vi "test_CSM.vi"(7 "Name (\"\" to Use UUID)":string="Event CSM Tiny") -> ()   [LabVIEW 2025]
doc: "Compact code template used to create a CSM module with a user interface. This template includes a user Event Structure for responding to user actions. The functionality of this template is identical to the CSM User Interface(UI) Module Template VI.\n\n\n> [!NOTE] <b>CSM Naming Rules</b>\n>\n> - CSM module name must be unique. Otherwise, CSM enters a `Critical Error` state.\n> - If the input module name is an empty string (\"\"), the system uses a UUID as the module name. Such a module is marked as standalone mode and does not appear in the module list.\n> - Worker Mode Rule: If the input module name ends with `#`, a worker mode node will be instantiated. Multiple worker mode nodes can form a worker mode module.\n> - Chain of Responsibility Mode Rule: If the input module name ends with `$` followed by a number, a chain of responsibility mode node will be instantiated. Multiple chain of responsibility mode nodes can form a chain of responsibility mode module.\n> - System-Level Module Rule: If the input module name starts with `.`, the module is a system-level module. Under default settings, such modules are not listed by the CSM - List Modules VI and are suitable for instantiating modules that run in the background.\n> - Submodule Rule: `.` is also allowed in a module name to separate the module name into multiple parts. CSM does not have strict rules for submodules. The `.` in the module name only marks the logical relationship between different modules. From an execution perspective, they are considered independent modules. The only difference is that you can obtain a list of logical submodules via the CSM - List Submodules VI.\n\n\n-- <b>Controls</b> --\n- <b>Name (\"\" to use UUID)</b>: CSM module name. Refer to <b>CSM Naming Rules</b> for module naming rules."
uses:
  <userlib>/_NEVSTOP/Communicable State Machine(CSM)/AdvanceAPI/CSM - Revert Arguments-Safe String.vi
  <userlib>/_NEVSTOP/Communicable State Machine(CSM)/_Shared/Trim Single-line Text.vi
  <userlib>/_NEVSTOP/Communicable State Machine(CSM)/AdvanceAPI/CSM - Break Down Multiple States String.vi
  <userlib>/_NEVSTOP/Communicable State Machine(CSM)/AdvanceAPI/CSM - Compact Multiple States.vi
  <userlib>/_NEVSTOP/Communicable State Machine(CSM)/AdvanceAPI/CSM - Make String Arguments Safe.vi
  <userlib>/_NEVSTOP/Communicable State Machine(CSM)/AdvanceAPI/CSM - Keywords.vi
  <userlib>/_NEVSTOP/Communicable State Machine(CSM)/Communicable State Machine.lvlib
panel:
  out "State History":string
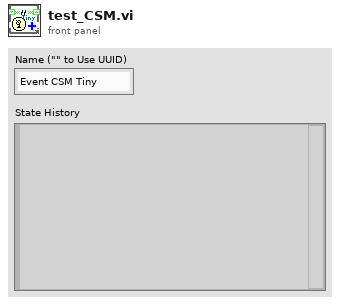
[diagram p1: front panel]
types:
  T1 = enum32{"Invalid", "Standard", "Closed", "Hidden", "Minimized", "Maximized"}
  T2 = enum32{"invalid app kind", "Development System", "Run Time System", "Student Edition", "Embedded LabVIEW", "Evaluation", "Custom"}
  T3 = typedef "Communicable State Machine.lvlib/_CSM_Response Source Message.ctl" = cluster{"‘State":string, "’Arguments":string, "’Error":errorcluster}
  T4 = cluster{"Current VI Reference":refnum<vi>, "Close Panel on Exit?":bool}
  T5 = cluster{"Core":cluster{"Current VI Reference":refnum<vi>, "Close Panel on Exit?":bool}, "Your Boolean data":bool, "Your string data":string}
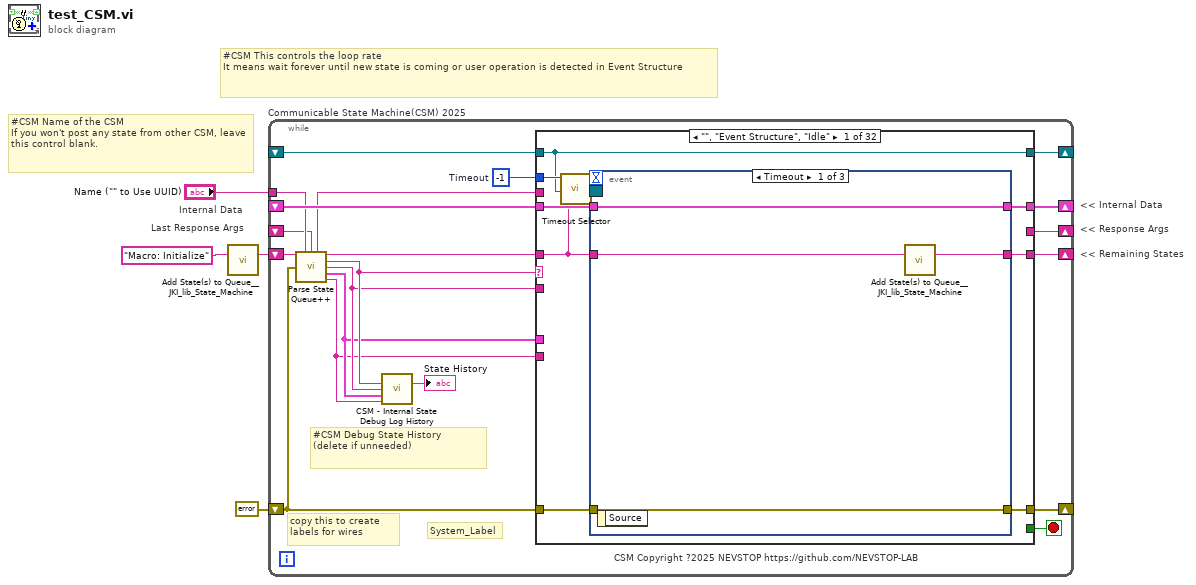
[diagram p0: block diagram]
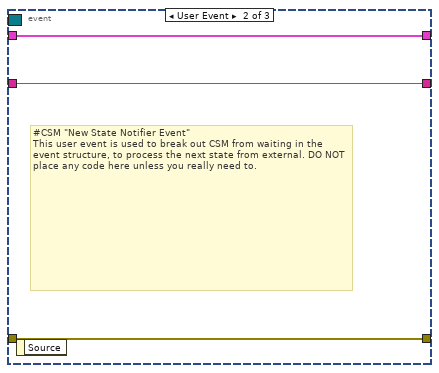
[diagram p2: hidden frame]
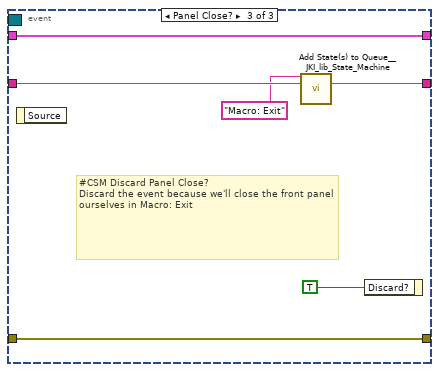
[diagram p3: hidden frame]
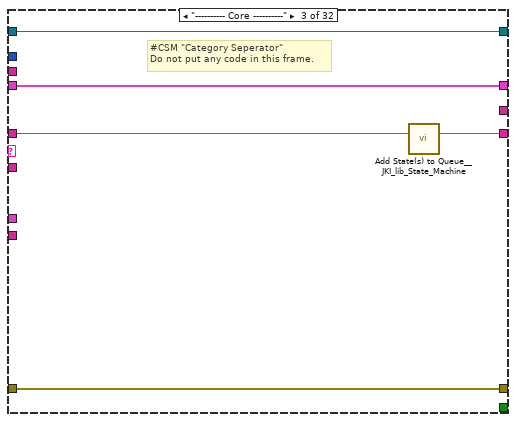
[diagram p5: hidden frame]
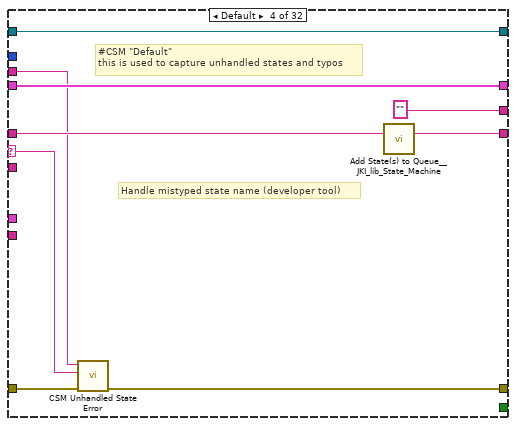
[diagram p6: hidden frame]
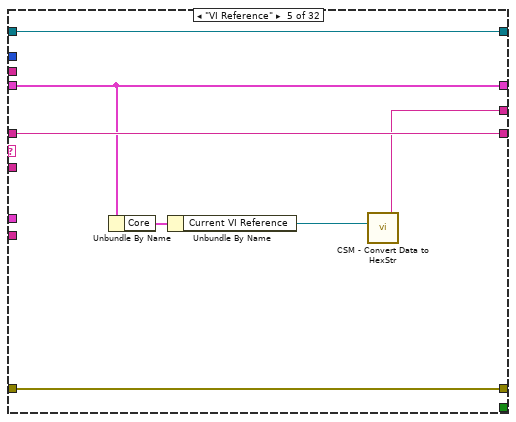
[diagram p7: hidden frame]
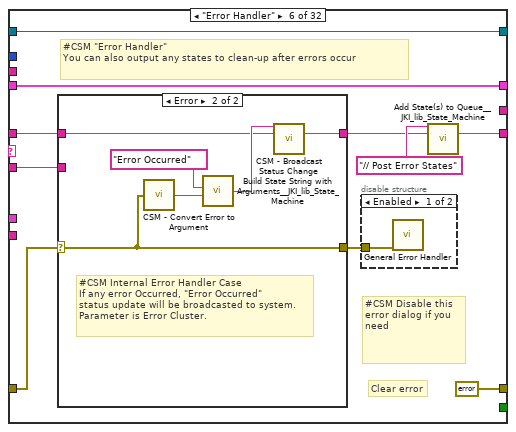
[diagram p8: hidden frame]
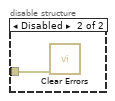
[diagram p9: hidden frame]
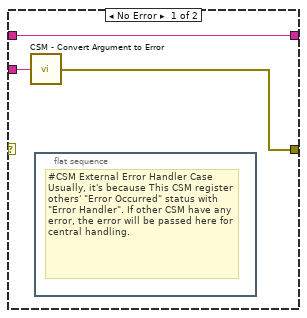
[diagram p10: hidden frame]
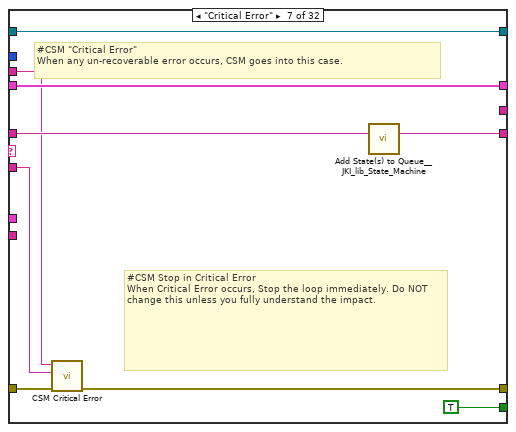
[diagram p11: hidden frame]
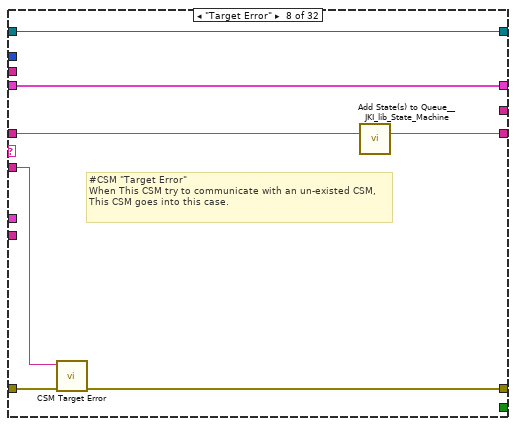
[diagram p12: hidden frame]
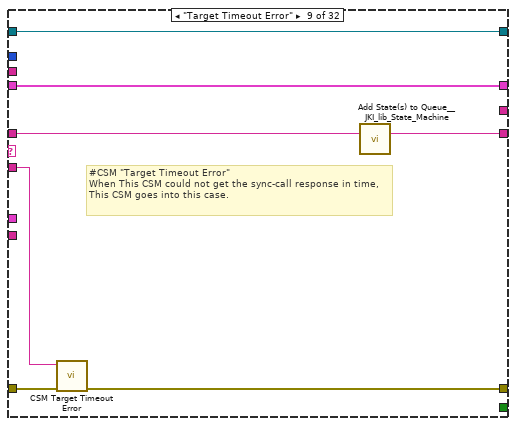
[diagram p13: hidden frame]
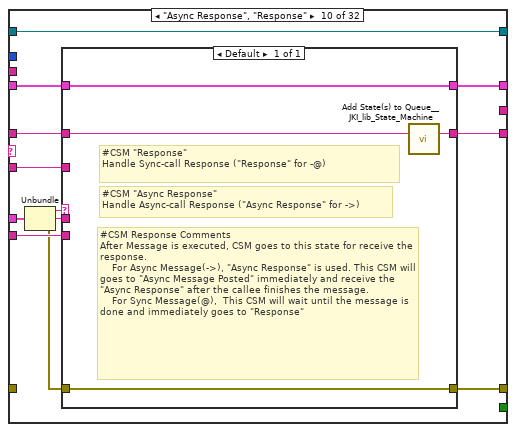
[diagram p14: hidden frame]
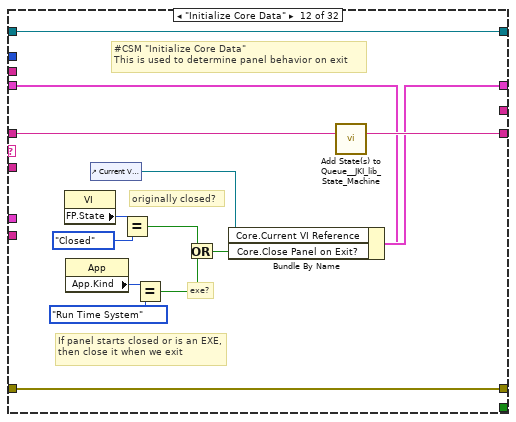
[diagram p16: hidden frame]
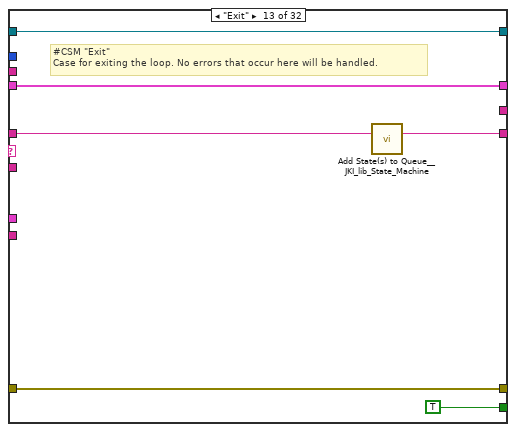
[diagram p17: hidden frame]
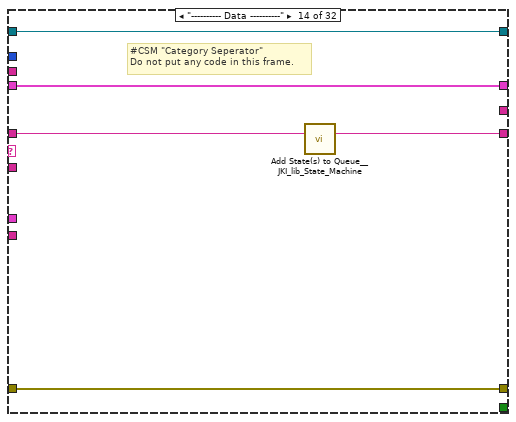
[diagram p18: hidden frame]
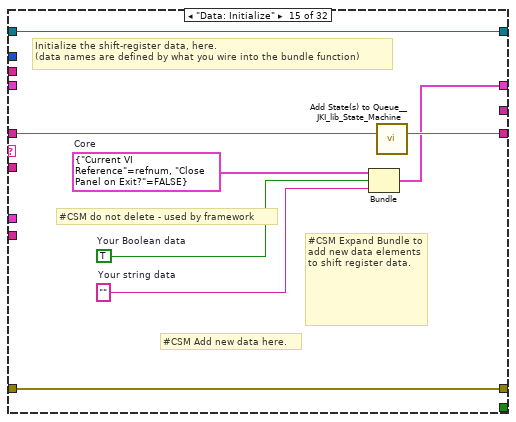
[diagram p19: hidden frame]
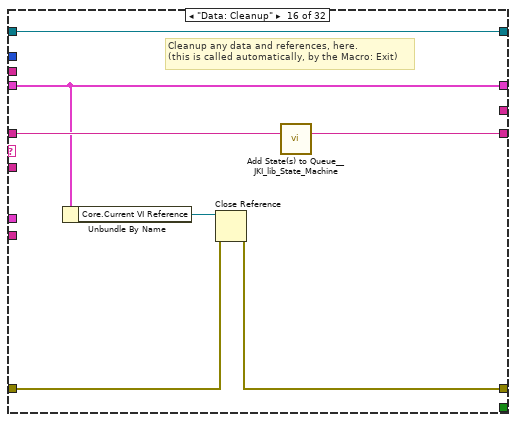
[diagram p20: hidden frame]
diagram:
  # "Last Response Args"
  # "Internal Data"
  # "#CSM Name of the CSM\nIf you won't post any state from other CSM, leave this control blank."
  # "#CSM This controls the loop rate\nIt means wait forever until new state is coming or user operation is detected in Event Structure"
  # "<< Internal Data"
  # "<< Response Args"
  # "<< Remaining States"
  n1 = call <vilib>:"Add State(s) to Queue__JKI_lib_State_Machine.vi"("State(s) in (\"\")"="Macro: Initialize" ("Init State(\"Macro: Initialize\")")) -> ("States Out"=w4:string)  [unwired: 14 in]
  n2 = while "Communicable State Machine(CSM) 2025" {
    shift-right: [w19] -> _
    shift-left: _ -> [w18]
    shift-right: [w22] -> _
    shift-left: errorcluster {"status"=FALSE, "code"=0, "source"=""} ("error out") -> [w16]
    shift-right: [w21] -> _
    shift-left: w4 -> [w23]
    tunnel: "Name (\"\" to Use UUID)" -> [w12]
    shift-right: [w15] -> _
    shift-left: _ -> [w6]
    shift-right: [w14] -> _
    shift-left: _ -> [w13]
    stop <- w20 stop-if-true
    w17 = -1  # Timeout
    # "#CSM Debug State History\n(delete if unneeded)"
    # "copy this to create labels for wires"
    # "System_Label"
    # "CSM Copyright ?2025 NEVSTOP https://github.com/NEVSTOP-LAB"
    n3 = call <userlib>:"Parse State Queue++.vi"("State Queue"=w23, "Name (\"\" to Use UUID)"=w12, "Response Arguments"=w6, "Previous Error"=w16) -> ("Name Used"=w7:string, "Remaining States"=w24:string, "Current State"=w11:string, "Arguments"=w10:string, "Additional Information"=w9:T3, "Source CSM"=w8:string)  [unwired: 6 in]
    n4 = call <userlib>:"CSM - Internal State Debug Log History.vi"("State"=w11, "Arguments (\"\")"=w10, ">> Response Source Message >>"=w9, "Source (\"\")"=w8) -> ("Debug Log"=→"State History":string)  [unwired: 11 in]
    n5 = case shown="\"\", \"Event Structure\", \"Idle\"" w11 {
      selector: w11 -> [_ _ _ w58 _ _ _ _ _ _ _ _ _ _ _ _ _ _ _ _ _ _ _ _ _ _ _ _ _ _ _ _]
      tunnel: w24 -> [w25 w49 w55 w63 w70 w76 w99 w105 w112 w121 w134 w149 w155 w160 w168 w175 w180 w187 w191 w197 w202 w209 w225 w295 w301 w313 w316 w321 w327 w335 w340 w345]
      tunnel: w10 -> [_ _ _ _ _ w75 w94 w104 w111 w120 _ _ _ _ _ _ _ _ _ _ _ w204 w219 _ _ _ _ _ w324 _ _ _]
      tunnel: w18 -> [w32 w48 w52 w61 w69 w80 w100 w107 w114 w123 w133 w142 w153 w157 _ w170 w177 w186 w190 w194 w200 w207 w221 w292 w298 w310 w315 w320 w326 w332 w337 w342]
      tunnel: [w31 w50 w53 w56 w71 errorcluster {"status"=FALSE, "code"=0, "source"=""} ("error out") w95 w102 w109 w126 w135 w146 w152 w158 w165 w171 w178 w181 w189 w195 w199 w205 w222 w293 w299 w311 w317 w322 w328 w333 w338 w343] -> w22
      tunnel: w16 -> [w30 w50 w53 w64 w71 w77 w101 w103 w110 _ w135 w146 w152 w158 w165 w172 w178 _ w192 w195 w199 w206 w223 w293 w299 w311 w317 w322 w328 w333 w338 w343]
      tunnel: [w33 w49 w54 w62 w70 w72 w98 w108 w115 w122 w134 w148 w154 w159 w167 w174 w179 w187 w191 w196 w201 w208 w224 w294 w300 w312 w316 w321 w327 w334 w339 w344] -> w21
      tunnel: [_ _ _ _ _ _ TRUE _ _ _ _ _ TRUE _ _ _ _ _ _ _ _ _ _ _ _ _ _ _ _ _ _ _] -> w20
      tunnel: [w29 w48 w52 w61 w69 w80 w100 w107 w114 w124 w133 w147 w153 w157 w166 w170 w177 w186 w190 w194 w200 w207 w221 w292 w298 w310 w315 w320 w326 w332 w337 w342] -> w19
      tunnel: w17 -> [w28 _ _ _ _ _ _ _ _ _ _ _ _ _ _ _ _ _ _ _ _ _ _ _ _ _ _ _ _ _ _ _]
      tunnel: w8 -> [_ _ _ _ _ _ _ _ _ w118 _ _ _ _ _ _ _ _ _ _ _ _ _ _ _ _ _ _ _ _ _ _]
      tunnel: w9 -> [_ _ _ _ _ _ _ _ _ w125 _ _ _ _ _ _ _ _ _ _ _ _ _ _ _ _ _ _ _ _ _ _]
      tunnel: [_ _ _ "" w65 _ _ _ _ _ _ _ _ _ _ _ _ _ _ _ _ _ _ _ _ _ _ "API1 Response" w323 _ _ _] -> w15
      tunnel: [w27 w47 w51 w59 w68 w79 w96 w106 w113 w127 w132 w136 w150 w156 w161 w169 w176 w185 w188 w193 w198 w203 w218 w291 w296 w303 w314 w319 w325 w331 w336 w341] -> w14
      tunnel: w13 -> [w27 w47 w51 w59 w68 w79 w96 w106 w113 w127 w132 w136 w150 w156 w161 w169 w176 _ w188 w193 w198 w203 w218 w291 w296 w303 w314 w319 w325 w331 w336 w341]
      tunnel: w7 -> [_ _ _ w57 _ _ w93 _ _ _ _ _ _ _ _ _ _ w184 _ _ _ _ _ _ _ _ _ _ _ _ _ _]
      frame "", "Event Structure", "Idle" {
        n6 = call <userlib>:"Timeout Selector.vi"("Remaining States"=w25, "Timeout Expected"=w28) -> ("Timeout"=w26:i32)  [unwired: 5 in]
        n7 = event shown="[0] Timeout" {
          selector: w27 -> [_ _ _]
          dyn-events: _ -> [_ _ _]
          timeout: w26 -> [_ _ _]
          tunnel: w25 -> [w37 w39 w46]
          tunnel: [w36 w39 w45] -> w33
          tunnel: w32 -> [w34 w40 w43]
          tunnel: [w35 w38 w44] -> w31
          tunnel: w30 -> [w35 w38 w44]
          tunnel: [w34 w40 w43] -> w29
          event Timeout {
            n8 = event-data() -> ()  [unwired: 1 in, 1 out]
            n9 = call <vilib>:"Add State(s) to Queue__JKI_lib_State_Machine.vi"("State(s) in (\"\")"=w37) -> ("States Out"=w36:string)  [unwired: 14 in]
          }
          event User Event {
            # "#CSM \"New State Notifier Event\"\nThis user event is used to break out CSM from waiting in the event structure, to process the next state from external. DO NOT place any code here unless you really need to."
            n10 = event-data() -> ()  [unwired: 1 in, 1 out]
          }
          event Panel Close? {
            # "#CSM Discard Panel Close?\nDiscard the event because we'll close the front panel ourselves in Macro: Exit"
            n11 = event-data() -> ()  [unwired: 1 in, 1 out]
            n12 = call <vilib>:"Add State(s) to Queue__JKI_lib_State_Machine.vi"("State(s) in Front (\"\")"="Macro: Exit", "State(s) in (\"\")"=w46) -> ("States Out"=w45:string)  [unwired: 13 in]
            n13 = event-data("Discard?"=TRUE) -> ()  [unwired: 1 in, 1 out]
          }
        }
      }
      frame "CSM Documentation" {
        # "#CSM README FIRST\n\nCommunicable State Machine(CSM) is a LabVIEW application framework that builds upon JKI State Machine(JKISM). It follows the pattern of JKISM and extends the keywords to describe message communication between modules, including concepts such as Sync-Message, Async-Message, Subscription/Unsubscription of status - essential elements for creating reusable code modules. For more information, please visit the CSM wiki: https://nevstop-lab.github.io/CSM-Wiki/\n\nFor instructions on JKI State Machine, visit: http://jki.net/state-machine/\nFor information about CSM, visit: https://github.com/NEVSTOP-LAB"
        # "#CSM \"Documentation\"\nCase for holding CSM Documenation"
      }
      frame "---------- Core ----------" {
        # "#CSM \"Category Seperator\"\nDo not put any code in this frame."
        n14 = call <vilib>:"Add State(s) to Queue__JKI_lib_State_Machine.vi"("State(s) in (\"\")"=w55) -> ("States Out"=w54:string)  [unwired: 14 in]
      }
      frame Default {
        # "#CSM \"Default\"\nthis is used to capture unhandled states and typos"
        # "Handle mistyped state name (developer tool)"
        n15 = call <userlib>:"CSM Unhandled State Error.vi"("error in (no error)"=w64, "Undefined State"=w58, "CSM Name"=w57) -> ("error out"=w56:errorcluster)  [unwired: 8 in]
        n16 = call <vilib>:"Add State(s) to Queue__JKI_lib_State_Machine.vi"("State(s) in (\"\")"=w63) -> ("States Out"=w62:string)  [unwired: 14 in]
      }
      frame "VI Reference" {
        n17 = Unbundle By Name(w69) -> ("Core"=w67:T4)
        n18 = Unbundle By Name(w67) -> ("Current VI Reference"=w66:refnum<vi>)
        n19 = call <userlib>:"CSM - Convert Data to HexStr.vi"("Variant"=w66) -> ("HEX String (0-9,A-F)"=w65:string)  [unwired: 8 in]
      }
      frame "Error Handler" {
        # "#CSM Disable this error dialog if you need"
        # "#CSM \"Error Handler\"\nYou can also output any states to clean-up after errors occur"
        # "Clear error"
        n20 = case shown="Error" w77 {
          selector: w77 -> [_ w87]
          tunnel: [w86 w89] -> w73
          tunnel: w76 -> [w86 w88]
          tunnel: w75 -> [w85 _]
          tunnel: [w84 w87] -> w78
          frame No Error {
            n21 = call <userlib>:"CSM - Convert Argument to Error.vi"("Argument"=w85) -> ("Error"=w84:errorcluster)  [unwired: 4 in]
            n22 = flat-sequence {
              frame #0 {
                # "#CSM External Error Handler Case\nUsually, it's because This CSM register others' \"Error Occurred\" status with \"Error Handler\". If other CSM have any error, the error will be passed here for central handling."
              }
            }
          }
          frame Error {
            # "#CSM Internal Error Handler Case \nIf any error Occurred, \"Error Occurred\" \nstatus update will be broadcasted to system.\nParameter is Error Cluster."
            n23 = call <userlib>:"CSM - Convert Error to Argument.vi"("Error"=w87) -> ("Argument"=w91:string)  [unwired: 4 in]
            n24 = call <vilib>:"Build State String with Arguments__JKI_lib_State_Machine.vi"("Arguments (\"\")"=w91, "State"="Error Occurred" ("Status with Arguments")) -> ("State with Arguments"=w90:string)  [unwired: 4 in]
            n25 = call <userlib>:"CSM - Broadcast Status Change.vi"("Status With Arguments"=w90, "State Queue"=w88) -> ("Remaining States"=w89:string)  [unwired: 13 in]
          }
        }
        n26 = disable-structure shown="Enabled" {
          disable-tunnel: w78 -> [w82 w83]
          frame Enabled {
            n27 = call <vilib>:"General Error Handler.vi"("error in (no error)"=w82) -> ()  [unwired: 10 in, 5 out]
          }
          frame Disabled {
            n28 = call <vilib>:"Clear Errors.vi"("error in (no error)"=w83) -> ()  [unwired: 5 in, 2 out]
          }
        }
        n29 = call <vilib>:"Add State(s) to Queue__JKI_lib_State_Machine.vi"("State(s) in Front (\"\")"="// Post Error States", "State(s) in (\"\")"=w73) -> ("States Out"=w72:string)  [unwired: 13 in]
      }
      frame "Critical Error" {
        # "#CSM Stop in Critical Error\nWhen Critical Error occurs, Stop the loop immediately. Do NOT change this unless you fully understand the impact."
        # "#CSM \"Critical Error\"\nWhen any un-recoverable error occurs, CSM goes into this case."
        n30 = call <userlib>:"CSM Critical Error.vi"("error in (no error)"=w101, "Arugments (As Reason)"=w94, "CSM Name"=w93) -> ("error out"=w95:errorcluster)  [unwired: 8 in]
        n31 = call <vilib>:"Add State(s) to Queue__JKI_lib_State_Machine.vi"("State(s) in (\"\")"=w99) -> ("States Out"=w98:string)  [unwired: 14 in]
      }
      frame "Target Error" {
        # "#CSM \"Target Error\"\nWhen This CSM try to communicate with an un-existed CSM, This CSM goes into this case."
        n32 = call <userlib>:"CSM Target Error.vi"("error in (no error)"=w103, "Arguments (As CSM Name)"=w104) -> ("error out"=w102:errorcluster)  [unwired: 9 in]
        n33 = call <vilib>:"Add State(s) to Queue__JKI_lib_State_Machine.vi"("State(s) in (\"\")"=w105) -> ("States Out"=w108:string)  [unwired: 14 in]
      }
      frame "Target Timeout Error" {
        # "#CSM \"Target Timeout Error\"\nWhen This CSM could not get the sync-call response in time, This CSM goes into this case."
        n34 = call <userlib>:"CSM Target Timeout Error.vi"("error in (no error)"=w110, "Arguments (As CSM Name)"=w111) -> ("error out"=w109:errorcluster)  [unwired: 9 in]
        n35 = call <vilib>:"Add State(s) to Queue__JKI_lib_State_Machine.vi"("State(s) in (\"\")"=w112) -> ("States Out"=w115:string)  [unwired: 14 in]
      }
      frame "Async Response", "Response" {
        n36 = Unbundle(w125) -> ("‘State"=w119:string, "’Arguments"=w117:string, "’Error"=w116:errorcluster)
        n37 = case shown="Default" w119 {
          tunnel: [w131] -> w126
          tunnel: w116 -> [w131]
          tunnel: [w130] -> w124
          tunnel: w123 -> [w130]
          tunnel: [w128] -> w122
          tunnel: w121 -> [w129]
          tunnel: w120 -> [_]
          tunnel: w118 -> [_]
          tunnel: w117 -> [_]
          frame Default {
            # "#CSM Response Comments\nAfter Message is executed, CSM goes to this state for receive the response.\n    For Async Message(->), \"Async Response\" is used. This CSM will goes to \"Async Message Posted\" immediately and receive the \"Async Response\" after the callee finishes the message.\n    For Sync Message(@),  This CSM will wait until the message is done and immediately goes to \"Response\""
            # "#CSM \"Async Response\"\nHandle Async-call Response (\"Async Response\" for ->)"
            # "#CSM \"Response\"\nHandle Sync-call Response (\"Response\" for -@)"
            n38 = call <vilib>:"Add State(s) to Queue__JKI_lib_State_Machine.vi"("State(s) in (\"\")"=w129) -> ("States Out"=w128:string)  [unwired: 14 in]
          }
        }
      }
      frame "Async Message Posted" {
        # "#CSM \"Async Message Posted\"\nAfter Async Message is posted (-> or ->| ), CSM goes to this state for post-action.\nYou can use Argument - State to tell which Async Message is called."
      }
      frame "Initialize Core Data" {
        # "#CSM \"Initialize Core Data\"\nThis is used to determine panel behavior on exit"
        # "originally closed?"
        # "exe?"
        # "If panel starts closed or is an EXE, then close it when we exit"
        n39 = property class="VI"() -> ("FP.State"=w139:T1)  [unwired: 2 in, 2 out]
        n40 = property class="App"() -> ("App.Kind"=w145:T2)  [unwired: 2 in, 2 out]
        n41 = control-ref of="Current VI Reference"() -> (w140:refnum<vi>)
        n42 = Equal?(x=w139, y=T1."Closed" ("Front Panel Window:State")) -> (x = y?=w137:bool)
        n43 = Equal?(x=w145, y=T2."Run Time System" ("Application:Kind")) -> (x = y?=w143:bool)
        n44 = Or(x=w137, y=w143) -> (x .or. y?=w141:bool)
        n45 = Bundle By Name(cluster=w142, "Core.Current VI Reference"=w140, "Core.Close Panel on Exit?"=w141) -> (w147:T5)
        n46 = call <vilib>:"Add State(s) to Queue__JKI_lib_State_Machine.vi"("State(s) in (\"\")"=w149) -> ("States Out"=w148:string)  [unwired: 14 in]
      }
      frame "Exit" {
        # "#CSM \"Exit\"\nCase for exiting the loop. No errors that occur here will be handled."
        n47 = call <vilib>:"Add State(s) to Queue__JKI_lib_State_Machine.vi"("State(s) in (\"\")"=w155) -> ("States Out"=w154:string)  [unwired: 14 in]
      }
      frame "---------- Data ----------" {
        # "#CSM \"Category Seperator\"\nDo not put any code in this frame."
        n48 = call <vilib>:"Add State(s) to Queue__JKI_lib_State_Machine.vi"("State(s) in (\"\")"=w160) -> ("States Out"=w159:string)  [unwired: 14 in]
      }
      frame "Data: Initialize" {
        w162 = T4 {"Current VI Reference"=refnum, "Close Panel on Exit?"=FALSE}  # Core
        w164 = TRUE  # Your Boolean data
        w163 = ""  # Your string data
        # "#CSM do not delete - used by framework"
        # "#CSM Expand Bundle to add new data elements to shift register data."
        # "#CSM Add new data here."
        # "Initialize the shift-register data, here.\n(data names are defined by what you wire into the bundle function)"
        n49 = Bundle("Core"=w162, "Your Boolean data"=w164, "Your string data"=w163) -> (w166:T5)  [unwired: 1 in]
        n50 = call <vilib>:"Add State(s) to Queue__JKI_lib_State_Machine.vi"("State(s) in (\"\")"=w168) -> ("States Out"=w167:string)  [unwired: 14 in]
      }
      frame "Data: Cleanup" {
        # "Cleanup any data and references, here.\n(this is called automatically, by the Macro: Exit)"
        n51 = Unbundle By Name(w170) -> ("Core.Current VI Reference"=w173:refnum<vi>)
        n52 = Close Reference(reference=w173, error in (no error)=w172) -> (error out=w171:errorcluster)
        n53 = call <vilib>:"Add State(s) to Queue__JKI_lib_State_Machine.vi"("State(s) in (\"\")"=w175) -> ("States Out"=w174:string)  [unwired: 14 in]
      }
      frame "---------- Events ----------" {
        # "#CSM \"Category Seperator\"\nDo not put any code in this frame."
        n54 = call <vilib>:"Add State(s) to Queue__JKI_lib_State_Machine.vi"("State(s) in (\"\")"=w180) -> ("States Out"=w179:string)  [unwired: 14 in]
      }
      frame "Events: Register" {
        # "#CSM \"Events: Register\"\nRegister user event. New Message Event is registered to break CSM waiting in event structure by default."
        # "#CSM Register New Message Event\nRegister message event to break Waiting in Event structure."
        n55 = call <userlib>:"CSM - Get New State Notifier Event.vi"("Name (\"\" to Use UUID)"=w184) -> ("error out"=w182:errorcluster, "New State Notifier Event"=w183:refnum<user-event>)  [unwired: 9 in]
        n56 = register-events(error in=w182, w183) -> (reference out=w185:refnum<event-registration>, error out=w181:errorcluster)  [unwired: 1 in]
      }
      frame "Events: Unregister" {
        # "#CSM \"Events: Unregister\"\nUnregister user event."
        n57 = Unregister For Events(event registration refnum=w188, error in=w192) -> (error out=w189:errorcluster)
      }
      frame "---------- UI ----------" {
        # "#CSM \"Category Seperator\"\nDo not put any code in this frame."
        n58 = call <vilib>:"Add State(s) to Queue__JKI_lib_State_Machine.vi"("State(s) in (\"\")"=w197) -> ("States Out"=w196:string)  [unwired: 14 in]
      }
      frame "UI: Initialize" {
        # "#CSM \"UI: Initialize\"\nInitialize the User Interface, here.\n(this is called automatically, by the Macro: Init)"
        n59 = call <vilib>:"Add State(s) to Queue__JKI_lib_State_Machine.vi"("State(s) in (\"\")"=w202) -> ("States Out"=w201:string)  [unwired: 14 in]
      }
      frame "UI: Cursor Set" {
        # "#CSM \"UI: Cursor Set\"\nSet and Unset Cursor Busy.\n(Usage: \"UI: Cursor Set >> Busy|Idle\")"
        # "Argument"
        n60 = disable-structure shown="Default" {
          disable-tunnel: w206 -> [w212 w217]
          disable-tunnel: [w211 w217] -> w205
          disable-tunnel: w204 -> [w210 _]
          frame condition #0 (active) {
            n61 = case shown="\"Idle\", Default" w210 {
              tunnel: w212 -> [w214 w216]
              tunnel: [w213 w215] -> w211
              frame "Idle", Default {
                n62 = call <vilib>:"Unset Busy.vi"("error in (no error)"=w214) -> ("error out"=w213:errorcluster)  [unwired: 10 in]
              }
              frame "Busy" {
                n63 = call <vilib>:"Set Busy.vi"("error in (no error)"=w216) -> ("error out"=w215:errorcluster)  [unwired: 9 in, 1 out]
              }
            }
          }
          frame condition #1 {
          }
        }
        n64 = call <vilib>:"Add State(s) to Queue__JKI_lib_State_Machine.vi"("State(s) in (\"\")"=w209) -> ("States Out"=w208:string)  [unwired: 14 in]
      }
      frame "UI: Front Panel State" {
        # "#CSM \"UI: Front Panel State\"\nSet Front Panel Open or Closed\n(Usage: \"UI: Front Panel State >> Open|Close\")"
        # "Argument"
        n65 = Unbundle By Name(w221) -> ("Core.Current VI Reference"=w220:refnum<vi>)
        n66 = call <vilib>:"Add State(s) to Queue__JKI_lib_State_Machine.vi"("State(s) in (\"\")"=w225) -> ("States Out"=w224:string)  [unwired: 14 in]
        n67 = case shown="\"Close\", \"Closed\"" w219 {
          tunnel: w223 -> [w231 w246 w257 w270 w283]
          tunnel: [w233 w247 w259 w272 w285] -> w222
          tunnel: w220 -> [w232 w244 w258 w271 w284]
          frame "Open", "Standard", Default {
            w226 = T1."Standard" ("State")
            n68 = property class="VI"(reference=w232, error in=w231) -> (reference out=w229:refnum<vi>, error out=w230:errorcluster, "FP.State"=w228:T1)
            n69 = Not Equal?(x=w228, y=w226) -> (x != y?=w227:bool)
            n70 = case shown="True" w227 {
              tunnel: [w237 w239] -> w233
              tunnel: w230 -> [w236 w239]
              tunnel: w229 -> [w235 _]
              tunnel: w226 -> [w234 _]
              frame True {
                n71 = invoke class="VI" method="FP.Open"(reference=w235, error in=w236, "Activate"=TRUE, "State"=w234) -> (error out=w237:errorcluster)  [unwired: 1 in, 4 out]
              }
              frame False {
              }
            }
          }
          frame "Close", "Closed" {
            n72 = property class="VI"(reference=w244, error in=w246) -> (reference out=w243:refnum<vi>, error out=w245:errorcluster, "FP.State"=w241:T1)
            n73 = Not Equal?(x=w241, y=T1."Closed" ("Front Panel Window:State")) -> (x != y?=w240:bool)
            n74 = case shown="False" w240 {
              tunnel: [w248 w251] -> w247
              tunnel: w245 -> [w248 w250]
              tunnel: w243 -> [_ w249]
              frame False {
              }
              frame True {
                n75 = invoke class="VI" method="FP.Close"(reference=w249, error in=w250) -> (error out=w251:errorcluster)  [unwired: 1 in, 2 out]
              }
            }
          }
          frame "Hidden", "Hide" {
            w252 = T1."Hidden" ("State")
            n76 = property class="VI"(reference=w258, error in=w257) -> (reference out=w255:refnum<vi>, error out=w256:errorcluster, "FP.State"=w254:T1)
            n77 = Not Equal?(x=w254, y=w252) -> (x != y?=w253:bool)
            n78 = case shown="True" w253 {
              tunnel: [w263 w264] -> w259
              tunnel: w256 -> [w262 w264]
              tunnel: w255 -> [w261 _]
              tunnel: w252 -> [w260 _]
              frame True {
                n79 = invoke class="VI" method="FP.Open"(reference=w261, error in=w262, "State"=w260) -> (error out=w263:errorcluster)  [unwired: 2 in, 4 out]
              }
              frame False {
              }
            }
          }
          frame "Minimize", "Minimized" {
            w265 = T1."Minimized" ("State")
            n80 = property class="VI"(reference=w271, error in=w270) -> (reference out=w268:refnum<vi>, error out=w269:errorcluster, "FP.State"=w267:T1)
            n81 = Not Equal?(x=w267, y=w265) -> (x != y?=w266:bool)
            n82 = case shown="True" w266 {
              tunnel: [w276 w277] -> w272
              tunnel: w269 -> [w275 w277]
              tunnel: w268 -> [w274 _]
              tunnel: w265 -> [w273 _]
              frame True {
                n83 = invoke class="VI" method="FP.Open"(reference=w274, error in=w275, "State"=w273) -> (error out=w276:errorcluster)  [unwired: 2 in, 4 out]
              }
              frame False {
              }
            }
          }
          frame "Maximize", "Maximized" {
            w278 = T1."Maximized" ("State")
            n84 = property class="VI"(reference=w284, error in=w283) -> (reference out=w281:refnum<vi>, error out=w282:errorcluster, "FP.State"=w280:T1)
            n85 = Not Equal?(x=w280, y=w278) -> (x != y?=w279:bool)
            n86 = case shown="True" w279 {
              tunnel: [w289 w290] -> w285
              tunnel: w282 -> [w288 w290]
              tunnel: w281 -> [w287 _]
              tunnel: w278 -> [w286 _]
              frame True {
                n87 = invoke class="VI" method="FP.Open"(reference=w287, error in=w288, "State"=w286) -> (error out=w289:errorcluster)  [unwired: 2 in, 4 out]
              }
              frame False {
              }
            }
          }
        }
      }
      frame "---------- Macro ----------" {
        # "#CSM \"Category Seperator\"\nDo not put any code in this frame."
        n88 = call <vilib>:"Add State(s) to Queue__JKI_lib_State_Machine.vi"("State(s) in (\"\")"=w295) -> ("States Out"=w294:string)  [unwired: 14 in]
      }
      frame "Macro: Initialize" {
        w297 = "Data: Initialize\nInitialize Core Data\nEvents: Register\nUI: Initialize\nUI: Front Panel State >> Open"  # Data: Initialize Initialize Core Data Events: Register UI: Initialize UI: Front Panel State >> Open
        # "#CSM \"Macro: Initialize\"\nInitialization Macro (This is called once, when the VI starts)"
        n89 = call <vilib>:"Add State(s) to Queue__JKI_lib_State_Machine.vi"("State(s) in Front (\"\")"=w297, "State(s) in (\"\")"=w301) -> ("States Out"=w300:string)  [unwired: 13 in]
      }
      frame "Macro: Exit" {
        # "#CSM \"Macro: Exit\"\nExit Macro (This is called once, when the VI exits)"
        n90 = Unbundle By Name(w310) -> ("Core.Close Panel on Exit?"=w309:bool)
        n91 = Select(t="UI: Front Panel State >> Close", s=w309, f="") -> (s? t:f=w306:string)
        n92 = call <vilib>:"Add State(s) to Queue__JKI_lib_State_Machine.vi"("State(s) in Front (\"\")"="//Exit Sub-Modules ", "State(s) in (\"\")"=w306, "State(s) at Back (\"\")"="Data: Cleanup\nEvents: Unregister\nExit") -> ("States Out"=w304:string)  [unwired: 12 in]
        n93 = call <vilib>:"Add State(s) to Queue__JKI_lib_State_Machine.vi"("State(s) in Front (\"\")"=w304, "State(s) in (\"\")"=w313) -> ("States Out"=w312:string)  [unwired: 13 in]
      }
      frame "---------- API ----------" {
        # "#CSM \"Category Seperator\"\nDo not put any code in this frame."
      }
      frame "API: API1" {
        # "#CSM API Example\nCopy/Rename this case for your own API"
        # "#CSM Response\nConnect this to return the response of your API"
        # "#CSM >> Source CSM >>\nIf you need to tell who triggered this state , use this string. If it's this case itself, this string is \"\"."
        # "#CSM >> Arguments >>\nDeal with the parameter if any"
      }
      frame "API: API2" {
        # "#CSM API Example\nCopy/Rename this case for your own API"
        # "unpack Hex String  to Variant\nif complex parameter is needed."
        n94 = call <userlib>:"CSM - Convert HexStr to Data.vi"("HEX String"=w324) -> ()  [unwired: 7 in, 2 out]
        n95 = disable-structure shown="Disabled" {
          disable-tunnel: [w329 "API2 Response"] -> w323
          frame Disabled {
            # "pack variant to hexstr \nif complex response is needed."
            # "complex Response"
            n96 = call <userlib>:"CSM - Convert Data to HexStr.vi"() -> ("HEX String (0-9,A-F)"=w329:string)  [unwired: 9 in]
          }
          frame Enabled {
          }
        }
      }
      frame "---------- Action ----------" {
        # "#CSM \"Category Seperator\"\nDo not put any code in this frame."
        n97 = call <vilib>:"Add State(s) to Queue__JKI_lib_State_Machine.vi"("State(s) in (\"\")"=w335) -> ("States Out"=w334:string)  [unwired: 14 in]
      }
      frame "Action: action1" {
        # "#CSM \"Internal State\"\nThis category is used for holding internal states"
        n98 = call <vilib>:"Add State(s) to Queue__JKI_lib_State_Machine.vi"("State(s) in (\"\")"=w340) -> ("States Out"=w339:string)  [unwired: 14 in]
      }
      frame "Action: action2" {
        # "#CSM \"Internal State\"\nThis category is used for holding internal states"
        n99 = call <vilib>:"Add State(s) to Queue__JKI_lib_State_Machine.vi"("State(s) in (\"\")"=w345) -> ("States Out"=w344:string)  [unwired: 14 in]
      }
    }
  }
